vi "Concatenate Multiple Fits.vi"(1 "Fits":T1(array[cluster])) -> (0 "Concatenated Fits":cluster{dbl[], dbl[]})   [LabVIEW 2013]
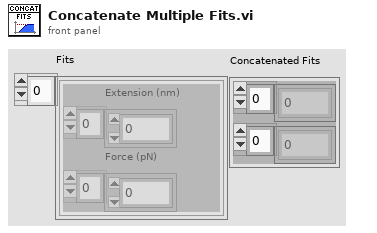
[diagram p1: front panel]
types:
  T1 = cluster{"Extension (nm)":dbl[], "Force (pN)":dbl[]}[]
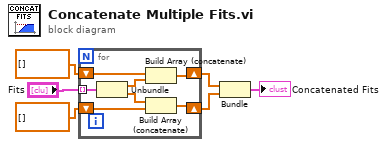
[diagram p0: block diagram]
diagram:
  n1 = for {
    tunnel: "Fits" -> [w13] mode=indexing
    shift-right: [w10] -> w5
    shift-left: dbl[] [] -> [w11]
    shift-right: [w8] -> w4
    shift-left: dbl[] [] -> [w9]
    n2 = Unbundle(w13) -> ("Extension (nm)"=w12:dbl[], "Force (pN)"=w7:dbl[])
    n3 = Build Array (concatenate)(w11, w12) -> (w10:dbl[])
    n4 = Build Array (concatenate)(w7, w9) -> (w8:dbl[])
  }
  n5 = Bundle(w5, w4) -> (→"Concatenated Fits":cluster{dbl[], dbl[]})  [unwired: 1 in]
